vi "Interpolate DBL Array.vi"(8 "Ending Value":dbl[](array[numeric]), 9 "Starting Value":dbl[](array[numeric]), 10 "Duration":dbl, 11 "Current Time":dbl) -> (3 "Current Value":dbl[](array[numeric]))   [LabVIEW 2018]
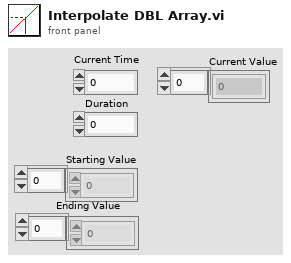
[diagram p1: front panel]
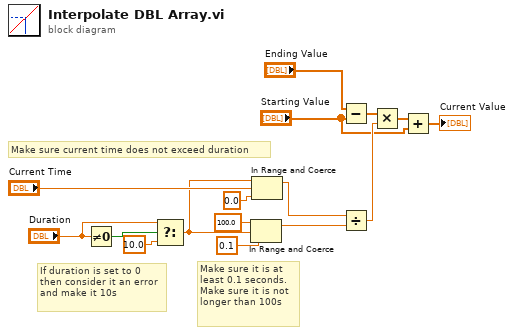
[diagram p0: block diagram]
diagram:
  # "Make sure it is at least 0.1 seconds.  Make sure it is not longer than 100s"
  # "Make sure current time does not exceed duration"
  # "If duration is set to 0 then consider it an error and make it 10s"
  n1 = Not Equal To 0?(x="Duration") -> (x != 0?=w10:bool)
  n2 = Select(t="Duration", s=w10, f=10.0) -> (s? t:f=w4:dbl)
  n3 = In Range and Coerce(upper limit=100.0, x=w4, lower limit=0.1) -> (coerced(x)=w3:dbl)  [unwired: 1 out]
  n4 = In Range and Coerce(upper limit=w4, x="Current Time", lower limit=0.0) -> (coerced(x)=w6:dbl)  [unwired: 1 out]
  n5 = Subtract(x="Ending Value", y="Starting Value") -> (x-y=w15:dbl[])
  n6 = Divide(x=w6, y=w3) -> (x/y=w14:dbl)
  n7 = Multiply(x=w15, y=w14) -> (x*y=w13:dbl[])
  n8 = Add(x=w13, y="Starting Value") -> (x+y=→"Current Value":dbl[])
